vi "Finalize To Settings.vi"(8 "error in (no error)":errorcluster, 11 "UDP Tx Transfer Configuration in":refnum<class "UDP Transfer Tx Configuration.lvclass">) -> (0 "error out":errorcluster, 2 "settings":cluster{"key":string, "value":string}[](array[cluster]), 3 "UDP Tx Transfer Configuration out":refnum<class "UDP Transfer Tx Configuration.lvclass">)   [LabVIEW 2017, in "UDP Transceiver.lvlib" / "UDP Transfer Tx Configuration.lvclass"]
uses:
  UDP Transfer Tx Configuration.lvclass
  UDP Transfer Tx Configuration.lvclass/UDP Transfer Tx Configuration.ctl
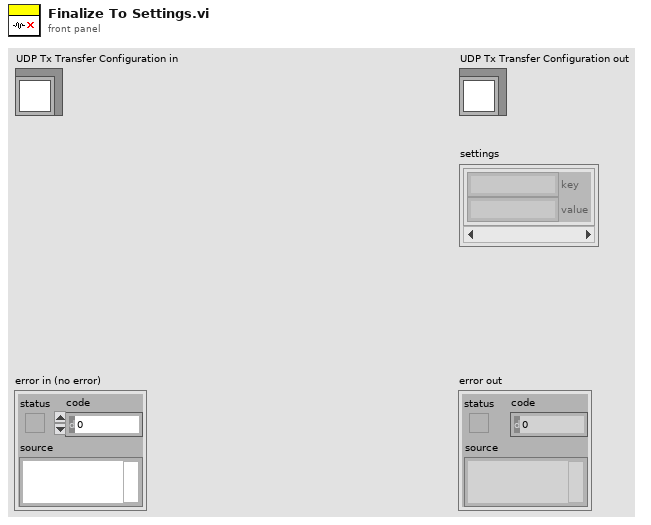
[diagram p1: front panel]
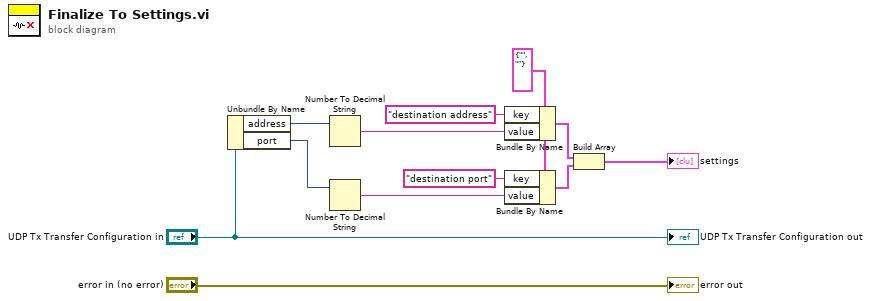
[diagram p0: block diagram]
diagram:
  w4 = cluster{"key":string, "value":string} {"key"="", "value"=""} ("setting")
  n1 = Unbundle By Name("UDP Tx Transfer Configuration in") -> ("address"=w6:u32, "port"=w5:u16)
  n2 = Number To Decimal String(number=w6) -> (decimal integer string=w12:string)  [unwired: 1 in]
  n3 = Number To Decimal String(number=w5) -> (decimal integer string=w7:string)  [unwired: 1 in]
  n4 = Bundle By Name(cluster=w4, "key"="destination address", "value"=w12) -> (w8:cluster{"key":string, "value":string})
  n5 = Bundle By Name(cluster=w4, "key"="destination port", "value"=w7) -> (w9:cluster{"key":string, "value":string})
  n6 = Build Array(w8, w9) -> (→"settings":cluster{"key":string, "value":string}[])
  "error out" <- "error in (no error)"
  "UDP Tx Transfer Configuration out" <- "UDP Tx Transfer Configuration in"
